vi "New.vi"(8 "error in (no error)":errorcluster, 11 "Observable in":refnum<class "Observable.lvclass">) -> (0 "error out":errorcluster, 3 "Observable out":refnum<class "Observable.lvclass">)   [LabVIEW 2011, in "Observable.lvclass"]
uses:
  Observable.lvclass
  Observer/Observer.lvclass
  Observable.lvclass/Observable.ctl
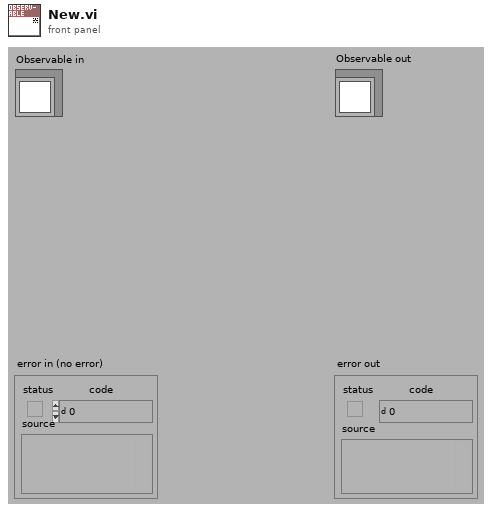
[diagram p1: front panel]
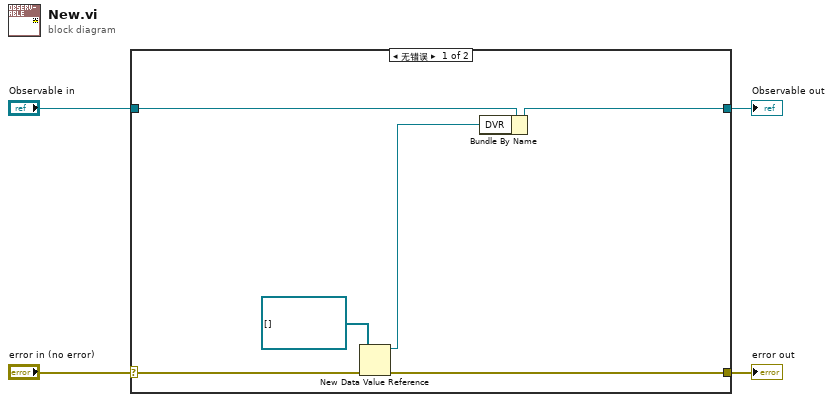
[diagram p0: block diagram]
diagram:
  n1 = case shown="无错误" "error in (no error)" {
    selector: "error in (no error)" -> [w10 w12]
    tunnel: [w7 w12] -> w1
    tunnel: [w8 w11] -> w3
    tunnel: "Observable in" -> [w9 w11]
    frame No Error {
      n2 = New Data Value Reference(data value=refnum<class "Observer.lvclass">[] [] ("Observers"), error in=w10) -> (data value reference=w6:refnum<data-value>, error out=w7:errorcluster)
      n3 = Bundle By Name(cluster=w9, "DVR"=w6) -> (w8:refnum<class "Observable.lvclass">)
    }
    frame Error {
    }
  }
  "Observable out" <- w3
  "error out" <- w1
